vi "LoadJSONVarSetIntoVM.vi"(8 "error in (no error)":errorcluster, 10 "JSONVarSet":T1, 11 "VariableManagerRef in":refnum<vi>) -> (0 "error out":errorcluster, 3 "VariableManagerRef out":refnum<vi>)   [LabVIEW 2013]
uses:
  VariableManagerCodes/VariableManager/VariableManager.lvclass
  JSONVarSet.ctl
  VariableManagerCodes/API/VariableManagerAPI.lvlib
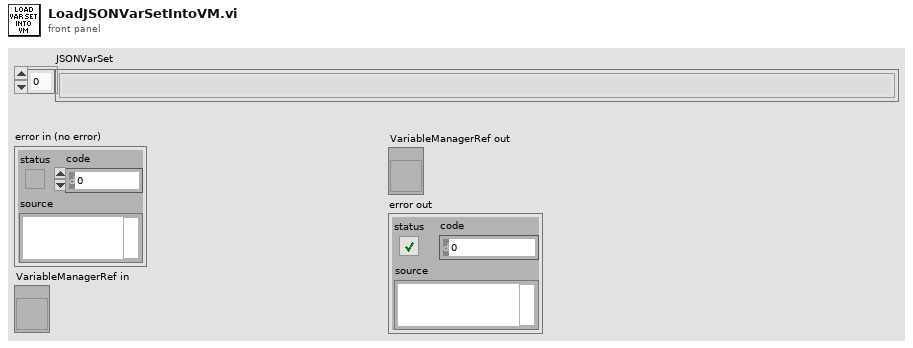
[diagram p1: front panel]
types:
  T1 = typedef "JSONVarSet.ctl" = string[]
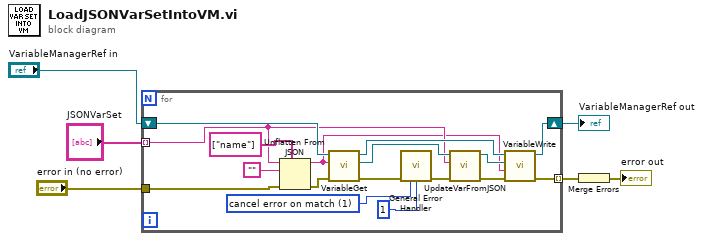
[diagram p0: block diagram]
diagram:
  n1 = for {
    shift-right: [w18] -> w4
    shift-left: "VariableManagerRef in" -> [w17]
    tunnel: "error in (no error)" -> [w8]
    tunnel: [w19] -> w3 mode=indexing
    tunnel: "JSONVarSet" -> [w10] mode=indexing
    w23 = 1 items=["no exception", "cancel error on match", "set error on match"] ("[exception action] (none:0)")
    n2 = Unflatten From JSON(path=string[] ["name"], JSON string=w10, type and defaults="", error in (no error)=w8) -> (value=w9:string, error out=w7:errorcluster)  [unwired: 3 in]
    n3 = call "VariableGet.vi"("error in (no error)"=w7, "VariableName"=w9, "VariableManagerRef in"=w17) -> ("error out"=w21:errorcluster, "Variable"=w16:refnum<class "Variable.lvclass">, "VariableManagerRef out"=w20:refnum<vi>)  [unwired: 6 in]
    n4 = call <vilib>:"General Error Handler.vi"("error in (no error)"=w21, "[exception action] (none:0)"=w23, "[exception code]"=1) -> ("error out"=w15:errorcluster)  [unwired: 8 in, 4 out]
    n5 = call "UpdateVarFromJSON.vi"("error in (no error)"=w15, "JSON Variable Object"=w10, "Variable.lvclass"=w16) -> ("error out"=w13:errorcluster, "reference out"=w14:refnum<class "Variable.lvclass">)  [unwired: 7 in]
    n6 = call "VariableWrite.vi"("error in (no error)"=w13, "OriginalName"=w9, "Variable"=w14, "VariableManagerRef in"=w20) -> ("error out"=w19:errorcluster, "VariableManagerRef out"=w18:refnum<vi>)  [unwired: 6 in]
  }
  "VariableManagerRef out" <- w4
  n7 = Merge Errors(w3) -> (→"error out":errorcluster)
